vi "profibus channel to string.vi"(11 "Profibus channel in":refnum<class "Profibus channel.lvclass">) -> (2 "channel data":string, 3 "identifier":string)   [LabVIEW 2013, in "Profibus channel.lvclass"]
uses:
  Profibus channel.lvclass
  <vilib>/NI/Tag Bus/tag/tag descriptor.lvclass/tag descriptor.ctl
  Profibus channel.lvclass/Profibus channel.ctl
  <vilib>/NI/Tag Bus Module Framework/channel/TBM channel.lvclass/TBM channel.ctl
  <vilib>/NI/Tag Bus/tag/tag descriptor.lvclass
  <vilib>/NI/Tag Bus Module Framework/channel/TBM channel.lvclass
  <vilib>/NI/Configuration Framework/serializable configuration/NISE_CEF_serializable configuration.lvclass
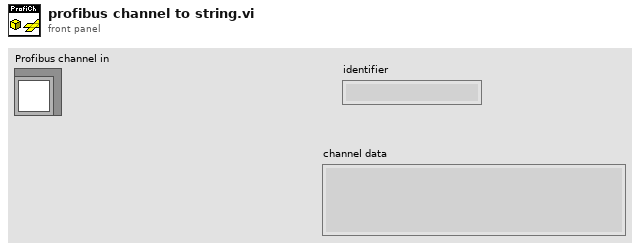
[diagram p1: front panel]
types:
  T1 = typedef "tag bus.lvlib/tag descriptor.lvclass/Data Type.ctl" = enum16{"Double", "Single", "I64", "I32", "I16", "I8", "U64", "U32", "U16", "U8", "Boolean", "String", "Array of Double", "Array of Single", "Array of I64", "Array of I32", "Array of I16", "Array of I8", "Array of U64", "Array of U32", "Array of U16", "Array of U8", "Array of Boolean", "Array of String"}
  T2 = typedef "TBM channel.lvclass/channel classification.ctl" = enum16{"input data", "output data", "processing parameter", "processing result"}
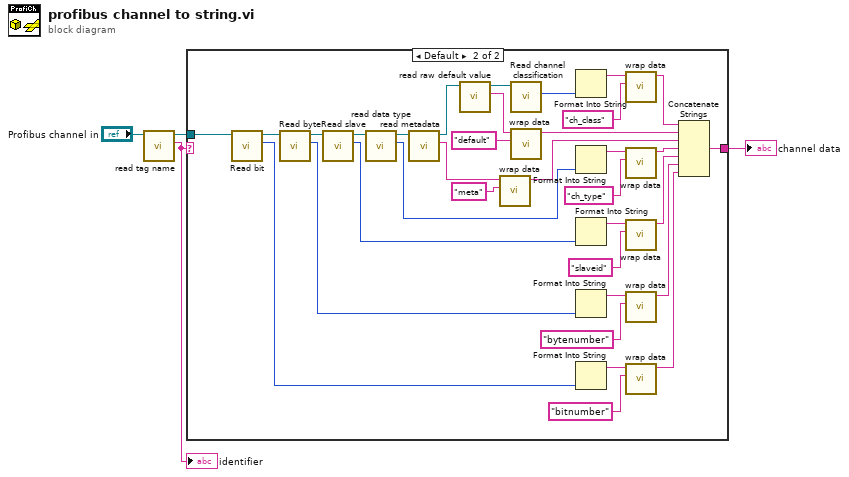
[diagram p0: block diagram]
diagram:
  n1 = call <vilib>:"read tag name.vi"("system tag in"="Profibus channel in") -> ("name"=w2:string, "system tag out"=w3:refnum<class "Profibus channel.lvclass">)  [unwired: 8 in, 1 out]
  "identifier" <- w2
  n2 = case shown="Default" w2 {
    selector: w2 -> [w5 _]
    tunnel: [w5 w22] -> w4
    tunnel: w3 -> [_ w13]
    frame "" {
    }
    frame Default {
      n3 = call "Read bit.vi"("Profibus channel in"=w13) -> ("bit"=w9:i32, "Profibus channel out"=w15:refnum<class "Profibus channel.lvclass">)  [unwired: 8 in, 1 out]
      n4 = call "Read byte.vi"("Profibus channel in"=w15) -> ("byte"=w10:i32, "Profibus channel out"=w14:refnum<class "Profibus channel.lvclass">)  [unwired: 8 in, 1 out]
      n5 = call "Read slave.vi"("Profibus channel in"=w14) -> ("slave"=w11:i8, "Profibus channel out"=w12:refnum<class "Profibus channel.lvclass">)  [unwired: 8 in, 1 out]
      n6 = call <vilib>:"read data type.vi"("system tag in"=w12) -> ("data type"=w37:T1, "system tag out"=w39:refnum<class "Profibus channel.lvclass">)  [unwired: 8 in, 1 out]
      n7 = call <vilib>:"read metadata.vi"("system tag in"=w39) -> ("metadata"=w32:string, "system tag out"=w38:refnum<class "Profibus channel.lvclass">)  [unwired: 8 in, 1 out]
      n8 = call <vilib>:"read raw default value.vi"("system tag in"=w38) -> ("raw default"=w31:string, "system tag out"=w34:refnum<class "Profibus channel.lvclass">)  [unwired: 8 in, 1 out]
      n9 = call <vilib>:"wrap data.vi"("identifier"="meta", "data to wrap"=w32) -> ("wrapped data"=w24:string)  [unwired: 9 in]
      n10 = call <vilib>:"Read channel classification.vi"("channel in"=w34) -> ("channel classification"=w29:T2)  [unwired: 8 in, 2 out]
      n11 = call <vilib>:"wrap data.vi"("identifier"="default", "data to wrap"=w31) -> ("wrapped data"=w25:string)  [unwired: 9 in]
      n12 = Format Into String(w29) -> (resulting string=w28:string)  [unwired: 3 in, 1 out]
      n13 = Format Into String(w37) -> (resulting string=w36:string)  [unwired: 3 in, 1 out]
      n14 = Format Into String(w11) -> (resulting string=w20:string)  [unwired: 3 in, 1 out]
      n15 = Format Into String(w10) -> (resulting string=w19:string)  [unwired: 3 in, 1 out]
      n16 = Format Into String(w9) -> (resulting string=w16:string)  [unwired: 3 in, 1 out]
      n17 = call <vilib>:"wrap data.vi"("identifier"="ch_class", "data to wrap"=w28) -> ("wrapped data"=w26:string)  [unwired: 9 in]
      n18 = call <vilib>:"wrap data.vi"("identifier"="ch_type", "data to wrap"=w36) -> ("wrapped data"=w23:string)  [unwired: 9 in]
      n19 = call <vilib>:"wrap data.vi"("identifier"="slaveid", "data to wrap"=w20) -> ("wrapped data"=w8:string)  [unwired: 9 in]
      n20 = call <vilib>:"wrap data.vi"("identifier"="bytenumber", "data to wrap"=w19) -> ("wrapped data"=w7:string)  [unwired: 9 in]
      n21 = call <vilib>:"wrap data.vi"("identifier"="bitnumber", "data to wrap"=w16) -> ("wrapped data"=w6:string)  [unwired: 9 in]
      n22 = Concatenate Strings(w26, w25, w24, w23, w8, w7, w6) -> (w22:string)
    }
  }
  "channel data" <- w4
